vi "CPC DAQ Example.vi"() -> ()   [LabVIEW 2014]
uses:
  CPC.lvclass
  Circular Buffer/1DSglBuffer/1D_Sgl_Buffer.lvclass
  <vilib>/Utility/file.llb/Write To Spreadsheet File (DBL).vi
  3022A/3022A.lvclass
  <vilib>/Utility/config.llb/NI_LVConfig.lvlib
  <vilib>/Utility/config.llb/Read Key (String).vi
  <vilib>/Utility/config.llb/Read Key (Path).vi
  <vilib>/Utility/config.llb/Read Key (I32).vi
  <vilib>/Platform/TimedLoop/XDataNode/XDataNode.xnode
  <vilib>/Platform/TimedLoop/XDataNode/nitl_modes.ctl
  <vilib>/Platform/TimedLoop/XDataNode/XDNodeRunTimeDep.lvlib
  <vilib>/Platform/TimedLoop/XDataNode/wakeup.ctl
  <vilib>/Platform/TimedLoop/XDataNode/timing_clust.ctl
  <vilib>/Utility/error.llb/DialogType.ctl
  DataClass/Array Data/Single 1-D/Single_Array.lvclass
  Controls/3022A/Flow.ctl
panel:
  out "On Time?":bool
  out "writing":bool
  in  "write":bool
  in  "Write Path":path
  out "CNc FP Concentration":cluster{"Time":timestamp[], sgl[]}(graph)
  in  "Flow Rate":T1
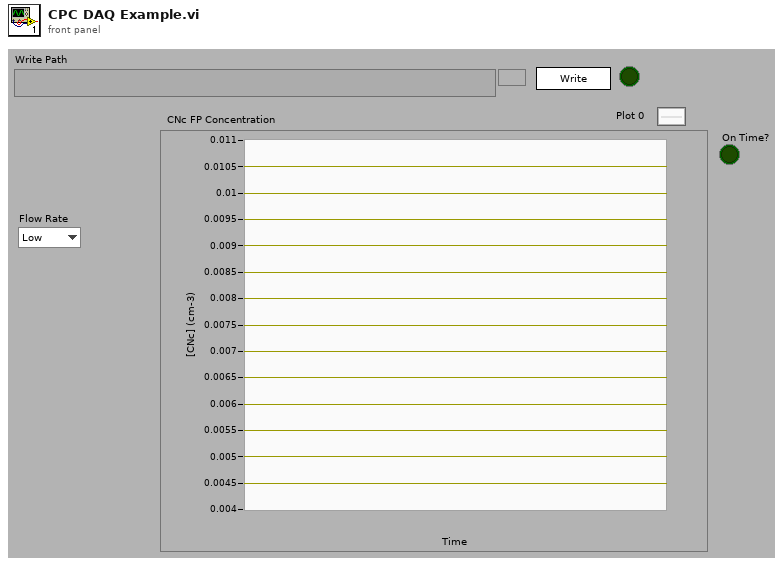
[diagram p1: front panel]
types:
  T1 = typedef "CPC.lvclass/Flow.ctl" = enum16{"Low", "High"}
  T2 = typedef "NI_LVConfig.lvlib/Config Data RefNum.ctl" = refnum<k1>
  T3 = typedef "XDNodeRunTimeDep.lvlib/timing_clust.ctl" = cluster{"Expected End [f-1]":u64, "Actual End [f-1]":u64, "Finished Late? [f-1]":bool, "Expected End [i-1]":u64, "Actual End [i-1]":u64, "Finished Late? [i-1]":bool, "Expected Start [i]":u64, "Actual Start [i]":u64, "Expected Start [f]":u64, "Actual Start [f]":u64, "Source Name":string, "Structure Name":string, "Period":i64, "Deadline":i64, "Offset":i64, "Start":i64, "Priority":i32, "Timeout":i32, "Mode":T4, "Wakeup Reason":T5, "Error":errorcluster, "Source Type":string, "Secondary Source Type":string, "Global End Time":u64, "Global Start Time":u64, "Frame Duration":u64, "Iteration Duration":u64, "Assigned CPU":i32, "I/O Scan Engine Mode":u32}
  T4 = typedef "XDNodeRunTimeDep.lvlib/nitl_modes.ctl" = enum32{"No Change", "Process missed periods, maintain original phase", "Discard missed periods, maintain original phase", "Process missed periods, ignore original phase", "Discard missed periods, ignore original phase"}
  T5 = typedef "XDNodeRunTimeDep.lvlib/wakeup.ctl" = enum32{"Normal", "Aborted", "Asynchronous wakeup", "Timing source error", "Timed loop error", "Timeout"}
  T6 = typedef "DialogType.ctl" = u16
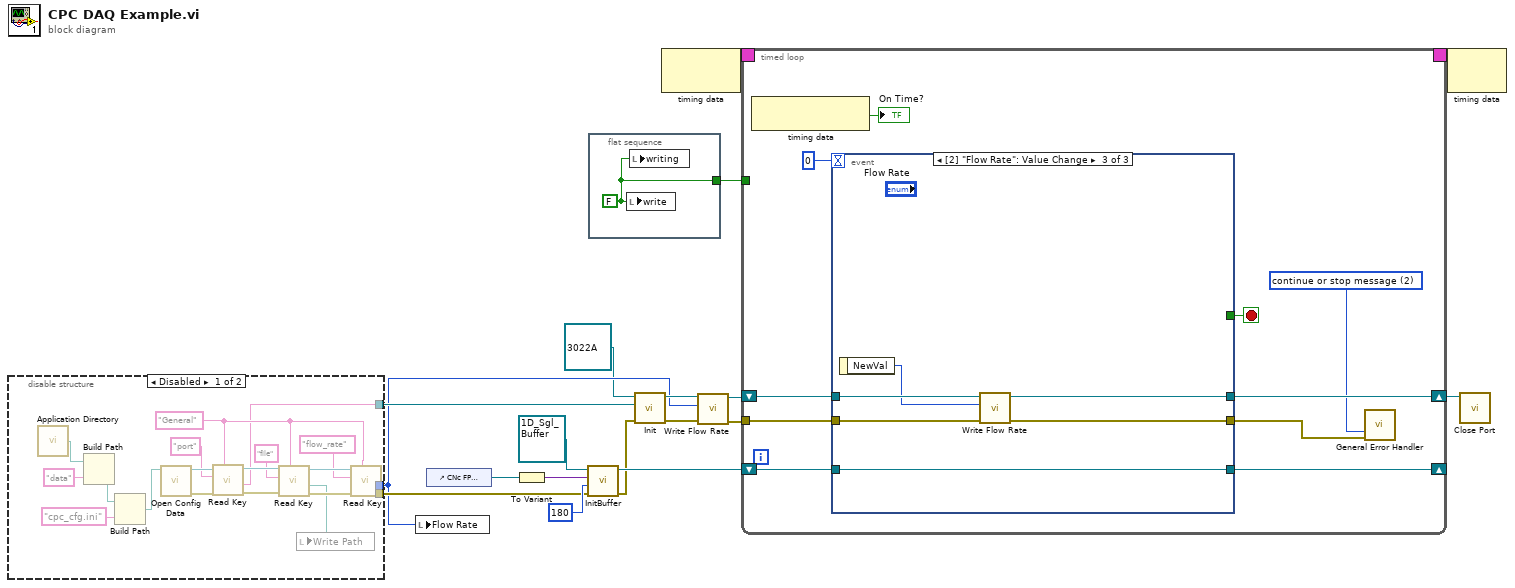
[diagram p0: block diagram]
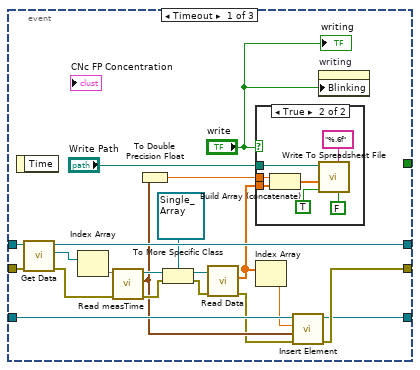
[diagram p3: hidden frame]
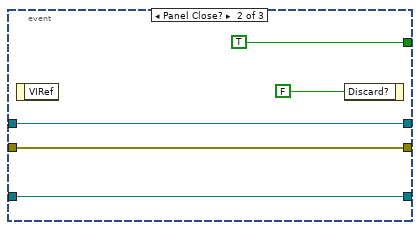
[diagram p5: hidden frame]
diagram:
  n1 = disable-structure shown="Disabled" {
    disable-tunnel: [w26 _] -> w9
    disable-tunnel: [w21 _] -> w8
    disable-tunnel: [w19 _] -> w3
    frame Disabled {
      w28 = "General" ("section")
      n2 = call <vilib>:"Application Directory.vi"() -> ("Application Directory"=w37:path)
      n3 = Build Path(base path=w37, name or relative path="data") -> (appended path=w25:path)
      n4 = Build Path(base path=w25, name or relative path="cpc_cfg.ini") -> (appended path=w24:path)
      n5 = call <vilib>:"Open Config Data.vi"("configuration file path"=w24) -> ("error out"=w35:errorcluster, "refnum"=w36:T2)  [unwired: 8 in, 1 out]
      n6 = call-poly <vilib>:"Read Key.vi"("section"=w28, "error in (no error)"=w35, "key"="port", "refnum"=w36) -> ("error out"=w32:errorcluster, "value"=w26:string, "refnum out"=w33:T2)  [unwired: 4 in, 1 out]
      n7 = call-poly <vilib>:"Read Key.vi"("section"=w28, "error in (no error)"=w32, "key"="file", "refnum"=w33) -> ("error out"=w29:errorcluster, "value"=w20:path, "refnum out"=w30:T2)  [unwired: 4 in, 1 out]
      n8 = local write "Write Path"(w20) -> ()
      n9 = call-poly <vilib>:"Read Key.vi"("section"=w28, "error in (no error)"=w29, "key"="flow_rate", "refnum"=w30) -> ("error out"=w21:errorcluster, "value"=w19:i32)  [unwired: 4 in, 2 out]
    }
    frame Enabled {
    }
  }
  n10 = local write "Flow Rate"(w3) -> ()
  n11 = control-ref of="CNc FP Concentration"() -> (w18:refnum<vi>)
  n12 = To Variant(anything=w18) -> (Variant=w17:variant)
  n13 = call-dynamic "InitBuffer.vi"("error in"=w8, "historyL"=u16 180, "GraphRef"=w17, "1D_Sgl_Buffer in"=refnum<class "1D_Sgl_Buffer.lvclass"> refnum ("1D_Sgl_Buffer.lvclass")) -> ("error out"=w7:errorcluster, "1D_Sgl_Buffer out"=w15:refnum<class "1D_Sgl_Buffer.lvclass">)  [unwired: 6 in]
  n14 = flat-sequence {
    tunnel: [w38] -> w2
    frame #0 {
      w38 = FALSE ("write")
      n15 = local write "write"(w38) -> ()
      n16 = local write "writing"(w38) -> ()
    }
  }
  n17 = call-dynamic "Init.vi"("error in (no error)"=w7, "Port"=w9, "3022A in"=refnum<class "3022A.lvclass"> refnum ("3022A.lvclass")) -> ("error out"=w12:errorcluster, "3022A out"=w13:refnum<class "3022A.lvclass">)  [unwired: 7 in]
  n18 = node-c288() -> (w6:T3)  [unwired: 1 in]
  n19 = call "Write Flow Rate.vi"("error in"=w12, "Flow Rate"=w3, "CPC in"=w13) -> ("error out"=w10:errorcluster, "CPC out"=w11:refnum<class "3022A.lvclass">)  [unwired: 7 in]
  n20 = timed-loop {
    tunnel: w10 -> [w47]
    shift-right: [w46] -> w4
    shift-left: w11 -> [w48]
    shift-right: [w44] -> _
    shift-left: w15 -> [w45]
    timing: w6 -> [_]
    timing-out: [_] -> w5
    tunnel: w2 -> [_]
    stop <- w39 stop-if-true
    w41 = T6 2 items=["no dialog", "OK message", "continue or stop message", "OK message + warnings", "continue/stop + warnings"] ("type of dialog (OK msg:1)")
    n21 = node-c288() -> (→"On Time?":bool)  [unwired: 1 in]
    n22 = event shown="[2] \"Flow Rate\": Value Change" {
      selector: _ -> [_ _ _]
      dyn-events: _ -> [_ _ _]
      timeout: 0 -> [_ _ _]
      tunnel: w48 -> [w71 w80 w89]
      tunnel: w47 -> [w70 w79 w88]
      tunnel: [w68 w80 w87] -> w46
      tunnel: [w65 w79 w86] -> w42
      tunnel: w45 -> [w67 w82 w85]
      tunnel: [_ TRUE ("Discard?") _] -> w39
      tunnel: [w59 w82 w85] -> w44
      event Timeout {
        n23 = event-data() -> ()  [unwired: 1 in, 1 out]
        n24 = call-dynamic "Get Data.vi"("error in"=w70, "CPC in"=w71) -> ("error out"=w61:errorcluster, "Data Out"=w69:refnum<class "CPC Data.lvclass">, "CPC out"=w68:refnum<class "3022A.lvclass">)  [unwired: 7 in]
        n25 = Index Array(array=w69) -> (element=w64)  [unwired: 1 in]
        n26 = call "Read measTime.vi"("error in (no error)"=w61, "Data in"=w64) -> ("error out"=w62:errorcluster, "measTime"=w60:timestamp, "Data out"=w63:refnum<class "Data.lvclass">)  [unwired: 7 in]
        n27 = To Double Precision Float(number=w60) -> (double precision float=w66:dbl)
        n28 = To More Specific Class(target class=refnum<class "Single_Array.lvclass"> refnum ("Single_Array.lvclass"), reference=w63, error in=w62) -> (specific class reference=w56:refnum<class "Single_Array.lvclass">, error out=w55:errorcluster)
        n29 = call "Read Data.vi"("error in (no error)"=w55, "Single_Array in"=w56) -> ("error out"=w54:errorcluster, "Data"=w52:sgl[])  [unwired: 7 in, 1 out]
        n30 = case shown="True" "write" {
          tunnel: w66 -> [_ w78]
          tunnel: "Write Path" -> [_ w73]
          tunnel: w52 -> [_ w72]
          frame False {
          }
          frame True {
            n31 = Build Array (concatenate)(w78, w72) -> (w77:dbl[])
            n32 = call-poly <vilib>:"Write To Spreadsheet File.vi"("transpose? (no:F)"=FALSE, "format (%.3f)"="%.6f", "append to file? (new file:F)"=TRUE, "1D data"=w77, "file path (dialog if empty)"=w73) -> ()  [unwired: 3 in, 1 out]
          }
        }
        n33 = Index Array(array=w52) -> (element=w53:sgl)  [unwired: 1 in]
        n34 = call "Insert Element.vi"("error in"=w54, "time"=w60, "data"=w53, "1D_Sgl_Buffer in"=w67) -> ("error out"=w65:errorcluster, "1D_Sgl_Buffer out"=w59:refnum<class "1D_Sgl_Buffer.lvclass">)  [unwired: 6 in]
        n35 = property on="writing" class="Bool (strict)"("Blinking"="write") -> ()  [unwired: 2 in, 2 out]
        "writing" <- "write"
      }
      event Panel Close? {
        n36 = event-data() -> ()  [unwired: 1 in, 1 out]
        n37 = event-data("Discard?"=FALSE) -> ()  [unwired: 1 in, 1 out]
      }
      event Value Change {
        n38 = event-data() -> ("NewVal"=w84:T1)  [unwired: 1 in]
        n39 = call "Write Flow Rate.vi"("error in"=w88, "Flow Rate"=w84, "CPC in"=w89) -> ("error out"=w86:errorcluster, "CPC out"=w87:refnum<class "3022A.lvclass">)  [unwired: 7 in]
      }
    }
    n40 = call <vilib>:"General Error Handler.vi"("type of dialog (OK msg:1)"=w41, "error in (no error)"=w42) -> ()  [unwired: 9 in, 5 out]
  }
  n41 = node-c288(w5) -> ()  [unwired: 1 out]
  n42 = call "Close Port.vi"("Serial IO in"=w4) -> ()  [unwired: 9 in, 2 out]
